vi "Init Unique GPIB.vi"(2 "Inited":u16[](array[numeric]), 3 "VISA resource name":refnum<visa-resource-name>) -> (0 "Inited dup":u16[](array[numeric]), 1 "dup VISA resource":refnum<visa-resource-name>)   [LabVIEW 2019]
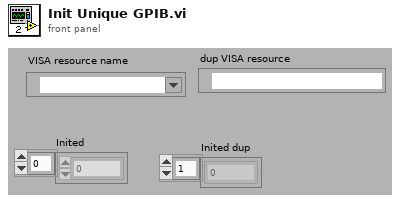
[diagram p1: front panel]
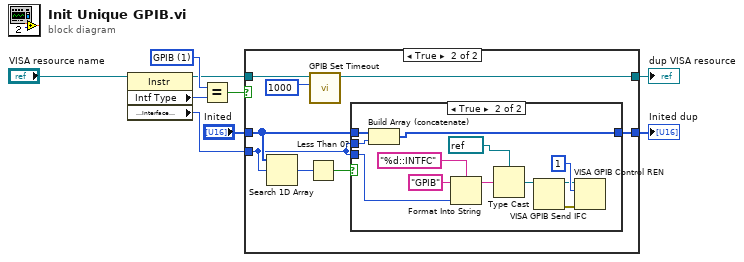
[diagram p0: block diagram]
diagram:
  w4 = u16 1 items=["GPIB"=1, "VXI"=2, "GPIB-VXI"=3, "Serial"=4, "PXI"=5, "TCPIP"=6, "USB"=7, "FireWire"=9] ("Interface Information:Interface Type")
  n1 = property class="Instr"(reference="VISA resource name") -> (reference out=w2:refnum<visa-resource-name>, "Intf Type"=w6:u16, "Interface Information:Interface Number"=w1:u16)  [unwired: 1 in, 1 out]
  n2 = Equal?(x=w4, y=w6) -> (x = y?=w5:bool)
  n3 = case shown="True" w5 {
    tunnel: w1 -> [_ w15]
    tunnel: "Inited" -> [w11 w16]
    tunnel: [w11 w17] -> w8
    tunnel: [w10 w13] -> w3
    tunnel: w2 -> [w10 w12]
    frame False {
    }
    frame True {
      n4 = Search 1D Array(1D array=w16, element=w15) -> (index of element=w19:i32)  [unwired: 1 in]
      n5 = Less Than 0?(x=w19) -> (x < 0?=w18:bool)
      n6 = call "GPIB Set Timeout.vi"("Timeout"=u32 1000 ("new timeout (10000)"), "VISA resource name"=w12) -> ("dup VISA resource name"=w13:refnum<visa-resource-name>)  [unwired: 3 in, 2 out]
      n7 = case shown="True" w18 {
        tunnel: [w20 w30] -> w17
        tunnel: w16 -> [w20 w32]
        tunnel: w15 -> [_ w31]
        tunnel: w15 -> [_ w26]
        frame False {
        }
        frame True {
          n8 = Build Array (concatenate)(w32, w31) -> (w30:u16[])
          n9 = Format Into String(format string="%d::INTFC", initial string="GPIB", w26) -> (resulting string=w25:string)  [unwired: 1 in, 1 out]
          n10 = Type Cast(type=refnum<visa-resource-name> refnum ("VISA resource name out"), x=w25) -> (*(type *) &x=w22:refnum<visa-resource-name>)
          n11 = VISA GPIB Send IFC(11:w22) -> (0:w24:errorcluster, 3:w23:refnum<visa-resource-name>)  [unwired: 1 in]
          n12 = VISA GPIB Control REN(8:w24, 10:u16 1 ("mode"), 11:w23) -> ()  [unwired: 2 out]
        }
      }
    }
  }
  "Inited dup" <- w8
  "dup VISA resource" <- w3
